vi "GE 5565PIORC.Memory.Read from DMA Block (DBL).vi"(8 "error in (no error)":errorcluster, 9 "count":u32, 10 "Block Descriptor in":T1 {"next descriptor ptr" format="%08x"; "data size" format="%08x"; "data ptr (upper)" format="%08x"; "data ptr (lower)" format="%08x"; "descriptor ptr (aligned)" format="%08x"; "descriptor size" format="%08x"; "descriptor ptr (VISA)" format="%08x"}, 11 "GE 5565PIORC in":refnum<class "GE 5565PIORC.lvclass">) -> (0 "error out":errorcluster, 1 "data out":dbl[](array[numeric]), 2 "Block Descriptor out":T1 {"next descriptor ptr" format="%08x"; "data size" format="%08x"; "data ptr (upper)" format="%08x"; "data ptr (lower)" format="%08x"; "descriptor ptr (aligned)" format="%08x"; "descriptor size" format="%08x"; "descriptor ptr (VISA)" format="%08x"}, 3 "GE 5565PIORC out":refnum<class "GE 5565PIORC.lvclass">)   [LabVIEW 2016, in "GE 5565PIORC.lvclass"]
doc: "Reads <B>count</B> elements from the provided <B>Block Descriptor</B> into a newly allocated <B>data</B> array."
uses:
  GE 5565PIORC.lvclass
  Typedefs/GE 5565PIORC.Typdef.DMA Block Descriptor.ctl
  GE 5565PIORC.lvclass/GE 5565PIORC.ctl
  <vilib>/Instr/_visa.llb/VISA Register Access Address Space.ctl
  GE 5565PIORC.Memory.VISA Return Handler.vi
  <vilib>/Utility/error.llb/Error Cluster From Error Code.vi
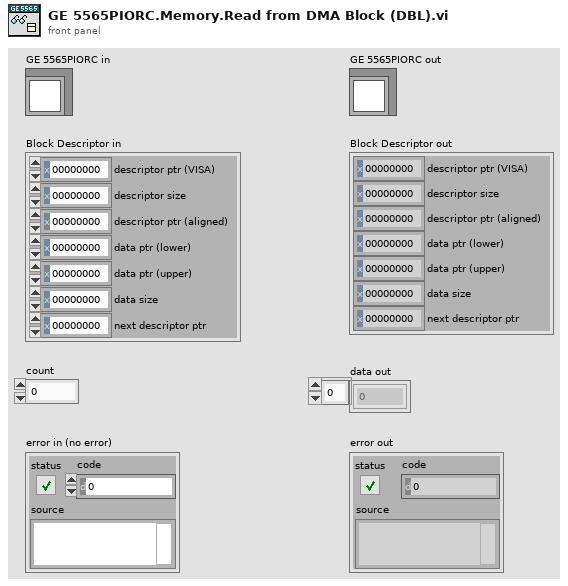
[diagram p1: front panel]
types:
  T1 = typedef "GE 5565PIORC.lvclass/GE 5565PIORC.Typdef.DMA Block Descriptor.ctl" = cluster{"descriptor ptr (VISA)":u32, "descriptor size":u32, "descriptor ptr (aligned)":u32, "data ptr (lower)":u32, "data ptr (upper)":u32, "data size":u32, "next descriptor ptr":u32}
  T2 = typedef "VISA Register Access Address Space.ctl" = u16
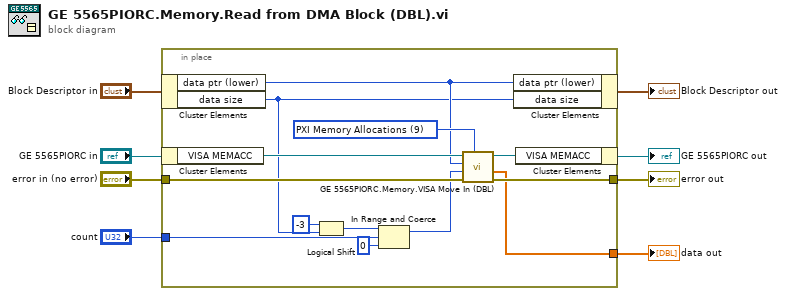
[diagram p0: block diagram]
diagram:
  n1 = in-place {
    in-place-border: "error in (no error)" -> [w18]
    in-place-border: [w19] -> w7
    in-place-border: "count" -> [w12]
    in-place-border: [w10] -> w1
    w16 = T2 9 items=["VXI/VME A16"=1, "VXI/VME A24"=2, "VXI/VME A32"=3, "VXI/VME A64"=4, "PXI Memory Allocations"=9, "PXI Configuration"=10, "PXI BAR0"=11, "PXI BAR1"=12, "PXI BAR2"=13, "PXI BAR3"=14, "PXI BAR4"=15, "PXI BAR5"=16] ("address space")
    n2 = in-place-cluster #1("Block Descriptor in") -> ("data ptr (lower)"=w15:u32, "data size"=w9:u32)
    n3 = in-place-cluster #2("GE 5565PIORC in") -> ("VISA MEMACC"=w17:refnum<visa-resource-name>)
    n4 = Logical Shift(y=i16 -3, x=w9) -> (x << y=w14:u32)
    n5 = In Range and Coerce(upper limit=w14, x=w12, lower limit=u32 0) -> (coerced(x)=w13:u32)  [unwired: 1 out]
    n6 = call "GE 5565PIORC.Memory.VISA Move In (DBL).vi"("address space"=w16, "error in (no error)"=w18, "count"=w13, "offset (0)"=w15, "VISA resource name"=w17) -> ("error out"=w19:errorcluster, "data out"=w10:dbl[], "VISA resource name out"=w20:refnum<visa-resource-name>)  [unwired: 4 in]
    n7 = in-place-cluster #1("data ptr (lower)"=w15, "data size"=w9) -> (→"Block Descriptor out":T1)
    n8 = in-place-cluster #2("VISA MEMACC"=w20) -> (→"GE 5565PIORC out":refnum<class "GE 5565PIORC.lvclass">)
  }
  "error out" <- w7
  "data out" <- w1
